vi "JSON Scalar Array To LV Array.vi"(8 "Error In":errorcluster, 11 "JSON Array":string) -> (0 "Error Out":errorcluster, 2 "Array Data":string[](array[string]), 3 "Array Name":string)   [LabVIEW 2011, in "LMH-Toolbox.lvlib" / "LMH-Scripting.lvlib"]
doc: "Parse JSON scalar array into array name and data elements."
uses:
  LMH-Scripting.lvlib
  <vilib>/regexp/Match Regular Expression.xnode
  Common/LMH-Common.lvlib
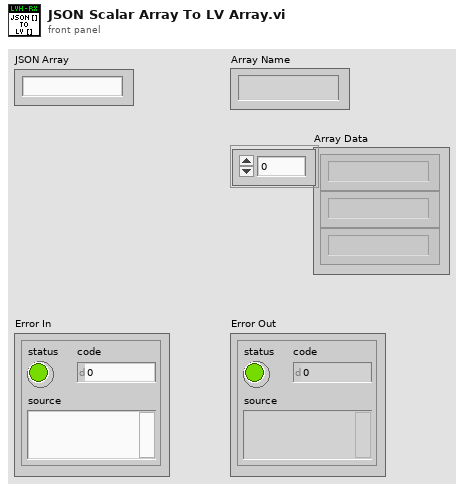
[diagram p1: front panel]
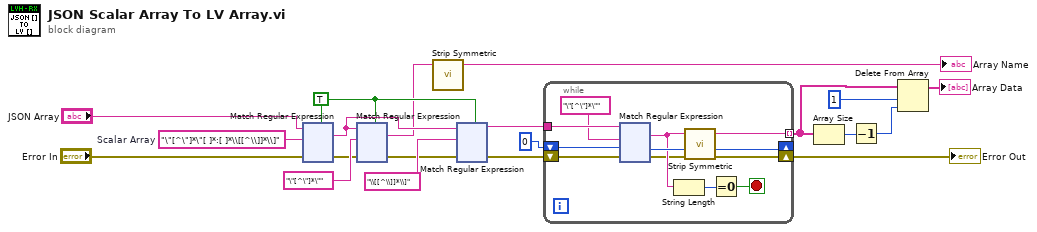
[diagram p0: block diagram]
diagram:
  w14 = TRUE ("multiline? (F)")
  w20 = "\"[^\"]*\"[ ]*:[ ]*\\[[^\\]]*\\]"  # Scalar Array
  n1 = xnode "Match Regular Expression"("input string"="JSON Array", "regular expression"=w20, "error in"="Error In", "multiline? (F)"=w14) -> ("whole match"=w18:string, "error out"=w16:errorcluster)  [unwired: 2 in, 3 out]
  n2 = xnode "Match Regular Expression"("input string"=w18, "regular expression"="\"[^\"]*\"", "error in"=w16, "multiline? (F)"=w14) -> ("whole match"=w10:string, "error out"=w15:errorcluster)  [unwired: 2 in, 3 out]
  n3 = call "Strip Symmetric.vi"("String"=w10) -> ("String"=→"Array Name":string)  [unwired: 4 in]
  n4 = xnode "Match Regular Expression"("input string"=w18, "regular expression"="\\[[^\\]]*\\]", "error in"=w15, "multiline? (F)"=w14) -> ("whole match"=w13:string, "error out"=w4:errorcluster)  [unwired: 2 in, 3 out]
  n5 = while {
    tunnel: w13 -> [w30]
    shift-right: [w27] -> _
    shift-left: 0 ("offset (0)") -> [w28]
    tunnel: [w23] -> w7 mode=indexing
    shift-right: [w21] -> w1
    shift-left: w4 -> [w22]
    stop <- w25 stop-if-true
    n6 = xnode "Match Regular Expression"("input string"=w30, "regular expression"="\"[^\"]*\"", "offset (0)"=w28, "error in"=w22) -> ("whole match"=w24:string, "offset past match"=w27:i32, "error out"=w21:errorcluster)  [unwired: 2 in, 2 out]
    n7 = String Length(string=w24) -> (length=w26:i32)
    n8 = call "Strip Symmetric.vi"("String"=w24) -> ("String"=w23:string)  [unwired: 4 in]
    n9 = Equal To 0?(x=w26) -> (x = 0?=w25:bool)
  }
  "Error Out" <- w1
  n10 = Array Size(array=w7) -> (size(s)=w5:i32)
  n11 = Decrement(x=w5) -> (x-1=w6:i32)
  n12 = Delete From Array(array=w7, length=1, index=w6) -> (array with subset deleted=→"Array Data":string[])  [unwired: 1 out]
